vi "Handle Error.vi"(8 "error in (no error)":errorcluster, 11 "Client Proxy LNA in":refnum<class "Client Proxy LNA.lvclass">) -> (0 "error out":errorcluster, 2 "stop actor?":bool=TRUE, 3 "Client Proxy LNA out":refnum<class "Client Proxy LNA.lvclass">)   [LabVIEW 2015, in "Client Proxy LNA.lvlib" / "Client Proxy LNA.lvclass"]
doc: "(<B>Filename</B>: Actor Framework.lvlib:Actor.lvclass:Handle Error.vi)\n\nDefines how the actor handles an error that occurred while processing a message.\n\nBy default, this method does nothing except stop the actor. This method also treats error code 43 (coming from <B>error in</B>) as a sign that the actor shut down normally. In this situation, the Handle Error method does not return the error on <B>error out</B>, meaning the actor's caller will not receive it. All other error codes will be returned on <B>error out</B>.\n\nA descendant class may override this method to change this behavior."
uses:
  Client Proxy LNA.lvclass
  <vilib>/ActorFramework/Actor/Actor.lvclass/Actor.ctl
  <userlib>/_OpenG.lib/error/error.llb/Filter Error Codes (Array)__ogtk.vi
  <vilib>/NI/Actors/Linked Network Actor/Linked Network Actor/Linked Network Actor.lvclass
  <userlib>/Common Components/Controller/Messages/Log Status/Log Status.lvclass
  <vilib>/ActorFramework/Actor/Actor.lvclass
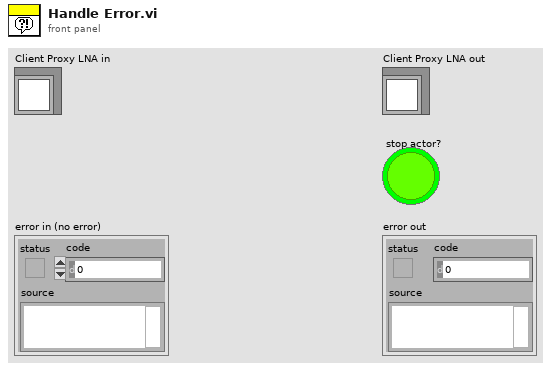
[diagram p1: front panel]
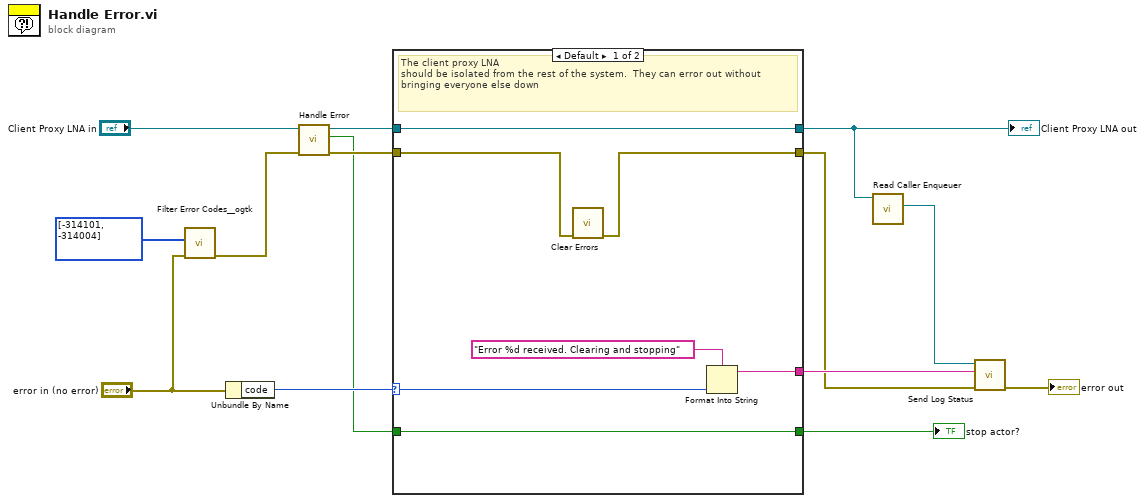
[diagram p0: block diagram]
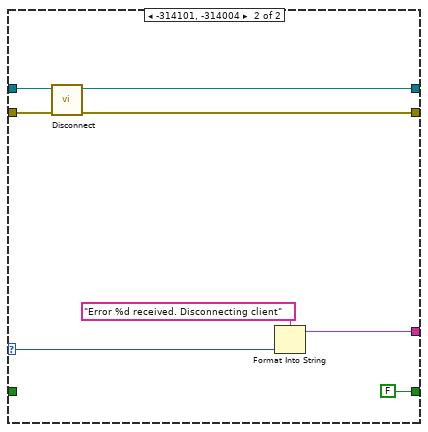
[diagram p2: hidden frame]
diagram:
  n1 = call-poly <userlib>:"Filter Error Codes__ogtk.vi"("Error In"="error in (no error)", "Error Codes to Filter"=i32[] [-314101, -314004]) -> ("Error Out"=w1:errorcluster)  [unwired: 7 in, 2 out]
  n2 = Unbundle By Name("error in (no error)") -> ("code"=w13:i32)
  n3 = call-parent "Handle Error.vi"("error in (no error)"=w1, "Linked Network Actor in"="Client Proxy LNA in") -> ("error out"=w6:errorcluster, "stop actor?"=w5:bool, "Linked Network Actor out"=w8:refnum<class "Client Proxy LNA.lvclass">)  [unwired: 7 in]
  n4 = case shown="Default" w13 {
    selector: w13 -> [w18 w27]
    tunnel: w5 -> [w21 _]
    tunnel: [w21 FALSE ("stop actor?")] -> w3
    tunnel: w8 -> [w20 w26]
    tunnel: [w20 w25] -> w4
    tunnel: w6 -> [w16 w24]
    tunnel: [w15 w23] -> w10
    tunnel: [w17 w22] -> w11
    frame Default {
      # "The client proxy LNA\nshould be isolated from the rest of the system.  They can error out without\nbringing everyone else down"
      n5 = call <vilib>:"Clear Errors.vi"("error in (no error)"=w16) -> ("error out"=w15:errorcluster)  [unwired: 5 in, 1 out]
      n6 = Format Into String(format string="Error %d received. Clearing and stopping" ("String"), w18) -> (resulting string=w17:string)  [unwired: 2 in, 1 out]
    }
    frame -314101, -314004 {
      n7 = call-dynamic "Disconnect.vi"("error in (no error)"=w24, "Network Actor in"=w26) -> ("error out"=w23:errorcluster, "Network Actor out"=w25:refnum<class "Client Proxy LNA.lvclass">)  [unwired: 8 in]
      n8 = Format Into String(format string="Error %d received. Disconnecting client" ("String"), w27) -> (resulting string=w22:string)  [unwired: 2 in, 1 out]
    }
  }
  "Client Proxy LNA out" <- w4
  "stop actor?" <- w3
  n9 = call <vilib>:"Read Caller Enqueuer.vi"("Actor"=w4) -> ("Caller Enqueuer"=w12:refnum<class "Message Enqueuer.lvclass">)  [unwired: 10 in]
  n10 = call <userlib>:"Send Log Status.vi"("error in (no error)"=w10, "String"=w11, "Message Enqueuer in"=w12) -> ("error out"=→"error out":errorcluster)  [unwired: 7 in, 1 out]
